vi "模字量AD输入统计结果.vi"   [LabVIEW 2010]
uses:
  全局量/自动测试结果.vi
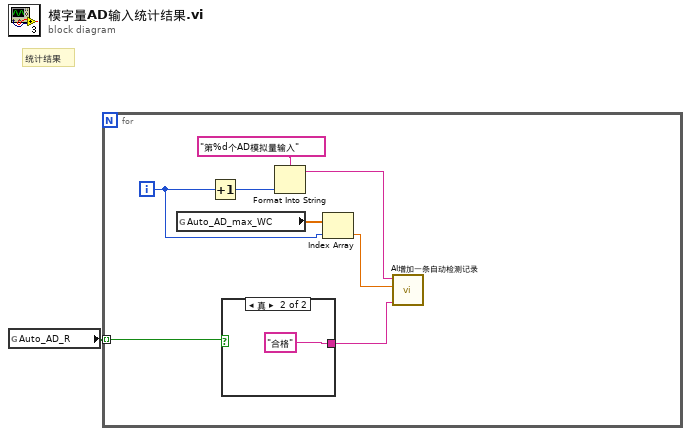
[diagram p0: block diagram]
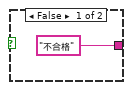
[diagram p2: hidden frame]
diagram:
  # "统计结果"
  n1 = global read "自动测试结果.vi" "Auto_AD_R"() -> (w1:bool[])
  n2 = for {
    tunnel: w1 -> [w9] mode=indexing
    i -> [w3]
    n3 = global read "自动测试结果.vi" "Auto_AD_max_WC"() -> (w4:dbl[])
    n4 = Increment(x=w3) -> (x+1=w8:i32)
    n5 = case shown="真" w9 {
      tunnel: ["不合格" "合格"] -> w5
      frame False {
      }
      frame True {
      }
    }
    n6 = Format Into String(format string="第%d个AD模拟量输入", w8) -> (resulting string=w6:string)  [unwired: 2 in, 1 out]
    n7 = Index Array(array=w4, index=w3) -> (element=w2:dbl)
    n8 = call "AI增加一条自动检测记录.vi"("测试结果"=w5, "最大误差"=w2, "测试内容"=w6) -> ()  [unwired: 9 in]
  }
